vi "Insight_Discovery_Decode.vi"(10 "IP Address (in)":string, 11 "IDN":string) -> (0 "Succeeded":bool, 2 "Serial Number":string, 3 "IP Address (out)":string)   [LabVIEW 2014]
panel:
  out "Model OK?":bool
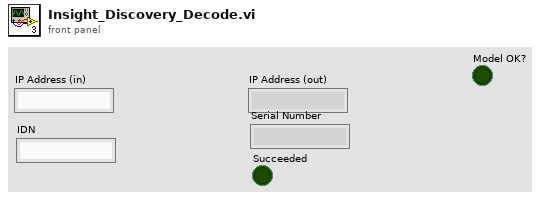
[diagram p1: front panel]
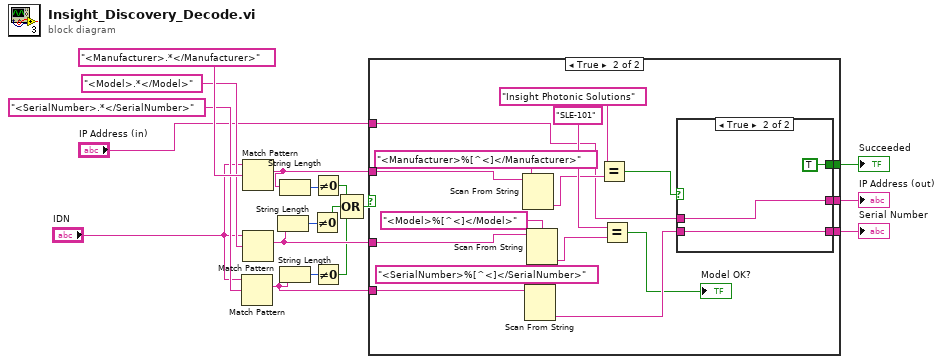
[diagram p0: block diagram]
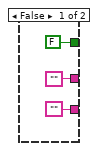
[diagram p2: hidden frame]
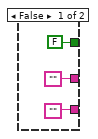
[diagram p3: hidden frame]
diagram:
  n1 = Match Pattern(string="IDN", regular expression="<SerialNumber>.*</SerialNumber>") -> (match substring=w6:string)  [unwired: 1 in, 3 out]
  n2 = Match Pattern(string="IDN", regular expression="<Manufacturer>.*</Manufacturer>") -> (match substring=w16:string)  [unwired: 1 in, 3 out]
  n3 = Match Pattern(string="IDN", regular expression="<Model>.*</Model>") -> (match substring=w15:string)  [unwired: 1 in, 3 out]
  n4 = String Length(string=w15) -> (length=w14:i32)
  n5 = String Length(string=w16) -> (length=w13:i32)
  n6 = String Length(string=w6) -> (length=w9:i32)
  n7 = Not Equal To 0?(x=w14) -> (x != 0?=w10:bool)
  n8 = Not Equal To 0?(x=w13) -> (x != 0?=w11:bool)
  n9 = Not Equal To 0?(x=w9) -> (x != 0?=w7:bool)
  n10 = Compound Arithmetic op=OR(w11, w10, w7) -> (w12:bool)
  n11 = case shown="True" w12 {
    tunnel: "IP Address (in)" -> [_ w31]
    tunnel: w16 -> [_ w33]
    tunnel: w15 -> [_ w32]
    tunnel: w6 -> [_ w28]
    tunnel: ["" w26] -> w5
    tunnel: ["" w25] -> w4
    tunnel: [FALSE ("Succeeded") w24] -> w1
    frame False {
    }
    frame True {
      n12 = Scan From String(format string="<Manufacturer>%[^<]</Manufacturer>" ("regular expression"), input string=w33) -> (output 1=w34:string)  [unwired: 3 in, 3 out]
      n13 = Scan From String(format string="<SerialNumber>%[^<]</SerialNumber>" ("regular expression"), input string=w28) -> (output 1=w27:string)  [unwired: 3 in, 3 out]
      n14 = Scan From String(format string="<Model>%[^<]</Model>" ("regular expression"), input string=w32) -> (output 1=w30:string)  [unwired: 3 in, 3 out]
      n15 = Equal?(x="Insight Photonic Solutions", y=w34) -> (x = y?=w23:bool)
      n16 = Equal?(x="SLE-101", y=w30) -> (x = y?=→"Model OK?":bool)
      n17 = case shown="True" w23 {
        tunnel: w31 -> [_ w44]
        tunnel: w27 -> [_ w43]
        tunnel: ["" w44] -> w26
        tunnel: ["" w43] -> w25
        tunnel: [FALSE ("Succeeded") TRUE ("Succeeded")] -> w24
        frame False {
        }
        frame True {
        }
      }
    }
  }
  "IP Address (out)" <- w5
  "Serial Number" <- w4
  "Succeeded" <- w1
